vi "Create (String Length).vi"(8 "error in (no error)":errorcluster, 9 "String length":i32, 10 "Number of strings":i32, 11 "String array in":string) -> (0 "error out":errorcluster, 3 "StringArray out":refnum<class "StringArray.lvclass">)   [LabVIEW 2013, in "MDSplus.lvlib" / "StringArray.lvclass"]
uses:
  <vilib>/MDSplus/Classes/Data_Class/Array_Class/StringArray_Class/StringArray.lvclass
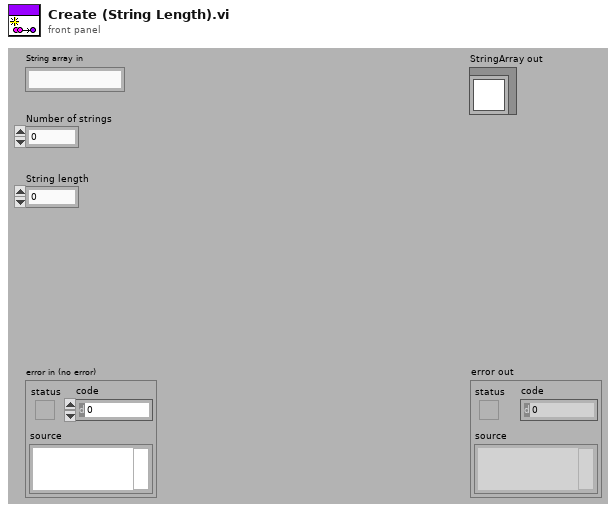
[diagram p1: front panel]
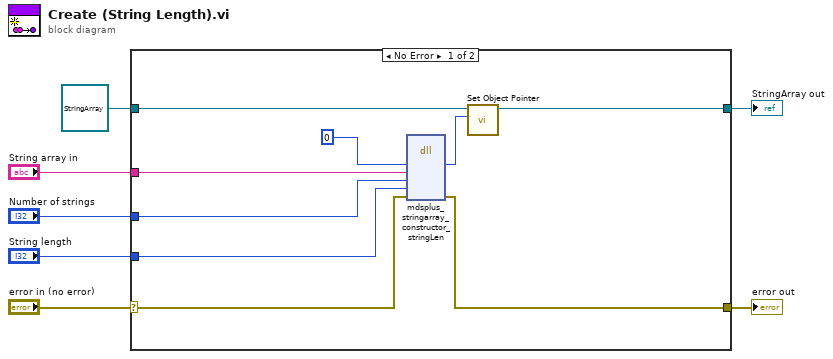
[diagram p0: block diagram]
diagram:
  n1 = case shown="No Error" "error in (no error)" {
    selector: "error in (no error)" -> [w14 w18]
    tunnel: [w10 w18] -> w6
    tunnel: [w12 w17] -> w4
    tunnel: refnum<class "StringArray.lvclass"> refnum ("Float32 in") -> [w13 w17]
    tunnel: "String array in" -> [w11 _]
    tunnel: "Number of strings" -> [w9 _]
    tunnel: "String length" -> [w8 _]
    frame No Error {
      n2 = dll-call lib="MDSobjectsLVShr" fn="mdsplus_stringarray_constructor_stringLen"("lvStringArrayPtrOut"=i64 0 ("lvTreePtr"), "dataIn"=w11, "nStringsIn"=w9, "stringLenIn"=w8, "error"=w14) -> ("lvStringArrayPtrOut"=w15:i64, "error"=w10:errorcluster)  [unwired: 7 in, 2 out]
      n3 = call-dynamic "Set Object Pointer.vi"("Object Pointer"=w15, "Data in"=w13) -> ("Data out"=w12:refnum<class "StringArray.lvclass">)  [unwired: 9 in]
    }
    frame Error {
    }
  }
  "error out" <- w6
  "StringArray out" <- w4
